vi "Orthogonize.vi"(2 "b":dbl[](array[numeric]), 3 "a":dbl[](array[numeric]) format="%#_13g", 4 "Theta2":dbl, 5 "Theta1":dbl) -> (0 "y":dbl[](array[numeric]), 1 "x":dbl[](array[numeric]))   [LabVIEW 2017]
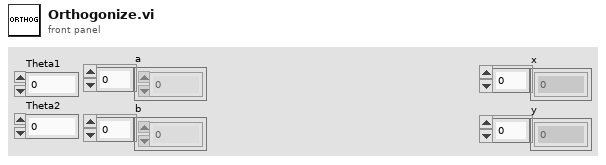
[diagram p1: front panel]
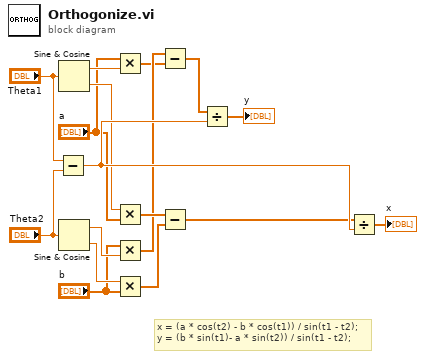
[diagram p0: block diagram]
diagram:
  # "x = (a * cos(t2) - b * cos(t1)) / sin(t1 - t2);\ny = (b * sin(t1)- a * sin(t2)) / sin(t1 - t2);"
  n1 = Subtract(x="Theta1", y="Theta2") -> (x-y=w17:dbl)
  n2 = Sine & Cosine(0:"Theta1") -> (1:w12:dbl, 2:w14:dbl)
  n3 = Sine & Cosine(0:"Theta2") -> (1:w10:dbl, 2:w13:dbl)
  n4 = Multiply(x="a", y=w12) -> (x*y=w5:dbl[])
  n5 = Multiply(x=w14, y="a") -> (x*y=w8:dbl[])
  n6 = Multiply(x="b", y=w10) -> (x*y=w6:dbl[])
  n7 = Multiply(x=w13, y="b") -> (x*y=w7:dbl[])
  n8 = Subtract(x=w6, y=w5) -> (x-y=w3:dbl[])
  n9 = Subtract(x=w8, y=w7) -> (x-y=w4:dbl[])
  n10 = Divide(x=w3, y=w17) -> (x/y=→"y":dbl[])
  n11 = Divide(x=w4, y=w17) -> (x/y=→"x":dbl[])
